vi "process.vi"(8 "error in":errorcluster, 11 "Data.PG":refnum<class "LV-Data.PGSQL.lvclass">) -> ()   [LabVIEW 2019, in "PGC2D.lvlib"]
uses:
  PGC2D.lvlib
  <userlib>/LevyLab/LV-Data/LV-Data.PG/LV-Data.PGSQL.lvclass
  sandbox/Instrument.AML.GetAll--Cluster.ctl
  typedefs/Instrument.AML.PGC2D_Chamber_ID--cluster.ctl
panel:
  in  "Log Fast":bool
  out "Prep Status 2":string caption="Status"
  out "Waveform Chart 2":dbl(graph)
  out "Waveform Chart":dbl(graph)
  out "Prep Current (A)":dbl=4.0 caption="Current (A)"
  out "Analysis Current (A)":dbl=2.0 caption="Current (A)"
  out "Prep Pirani (mbar) 1":dbl=7.0 caption="Pirani 1 (mbar)"
  out "Prep Pirani (mbar) 2":dbl=8.0 caption="Pirani 2 (mbar)"
  out "Analysis Pirani (mbar) 2":dbl=6.0 caption="Pirani 2 (mbar)"
  out "Analysis Pirani (mbar) 1":dbl=5.0 caption="Pirani 1 (mbar)"
  out "Prep Status":string caption="Status"
  out "Analysis Status":string caption="Status"
  out "state":string
  out "logger timer (ms)":u32
  out "Prep Pressure (mbar)":dbl=3.0 caption="IG (mbar)" format="%_2g"
  out "Analysis Pressure (mbar)":dbl=1.0 caption="IG (mbar)" format="%_2g"
  out "Data.PG out":refnum<class "LV-Data.PGSQL.lvclass">
  out "read timer (ms)":u32
  out "error out":errorcluster
  # "Analysis Chamber"
  # "Preparation Chamber"
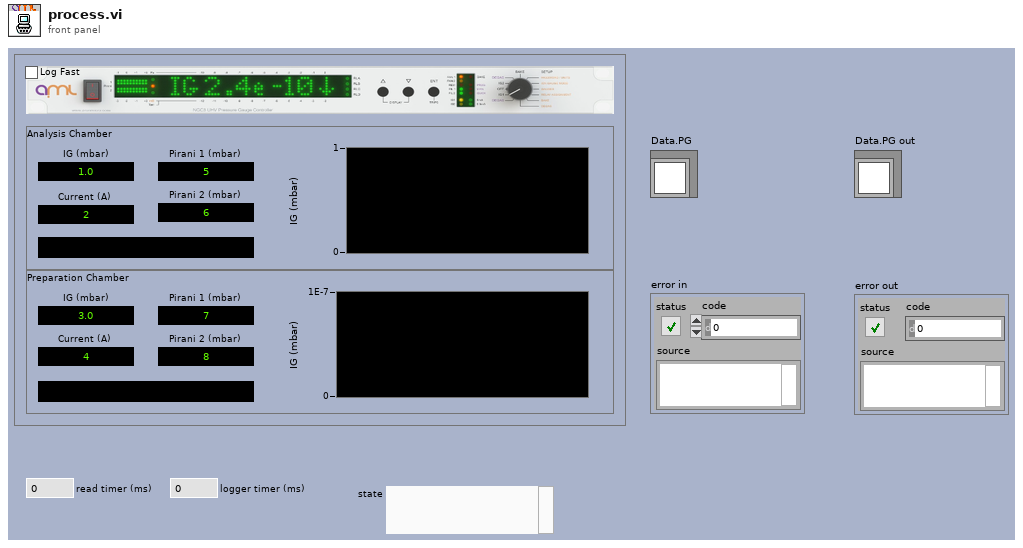
[diagram p1: front panel]
types:
  T1 = enum32{"Invalid", "Standard", "Closed", "Hidden", "Minimized", "Maximized"}
  T2 = enum32{"invalid app kind", "Development System", "Run Time System", "Student Edition", "Embedded LabVIEW", "Evaluation", "Custom"}
  T3 = typedef "PGC2D.lvlib/Instrument.AML.PGC2D_Chamber_ID--cluster.ctl" = cluster{"name":string, "Address":refnum<visa-resource-name>}
  T4 = typedef "Instrument.AML.GetAll--Cluster.ctl" = cluster{"IG Pressure (mbar)":dbl, "Pirani 1 Pressure (mbar)":dbl, "Pirani 2 Pressure (mbar)":dbl, "Emission Current (A)":dbl, "Trip A Pressure (mbar)":dbl, "Trip B Pressure (mbar)":dbl, "Trip C Pressure (mbar)":dbl, "Trip D Pressure (mbar)":dbl, "Instrument Status":string, "Fault":string, "Trip A Association":string, "Trip B Association":string, "Trip C Association":string, "Trip D Association":string, "Relay A":string, "Relay B":string, "Relay C":string, "Relay D":string}
  T5 = cluster{"Core":cluster{"Current VI Reference":refnum<vi>, "Close Panel on Exit?":bool}, "Data.PG":refnum<class "LV-Data.PGSQL.lvclass">, "Chamber ID":T3[], "AML cluster array":T4[]}
  T6 = cluster{"Current VI Reference":refnum<vi>, "Close Panel on Exit?":bool}
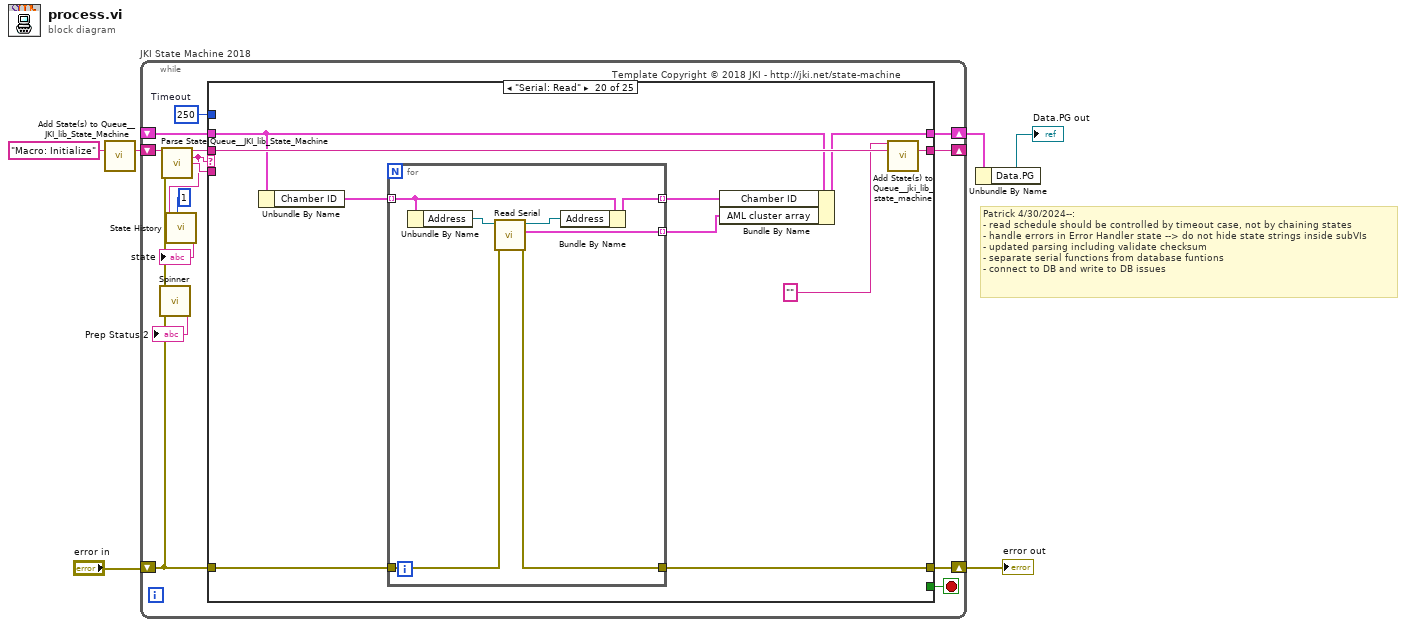
[diagram p0: block diagram]
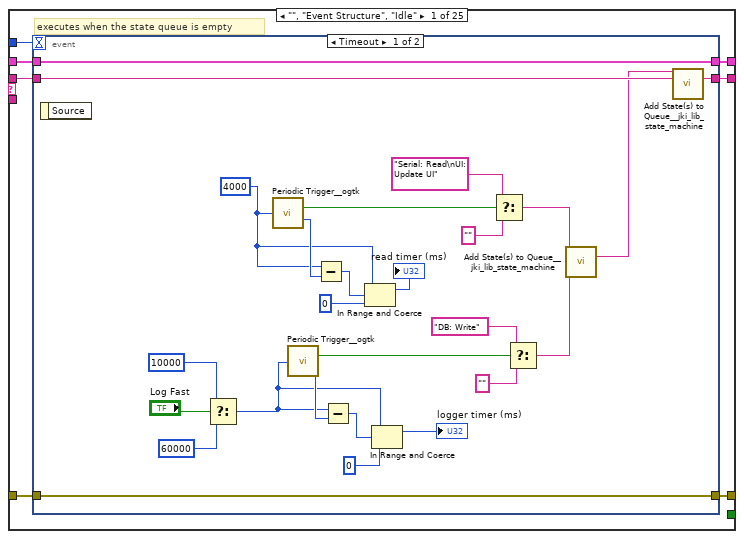
[diagram p2: hidden frame]
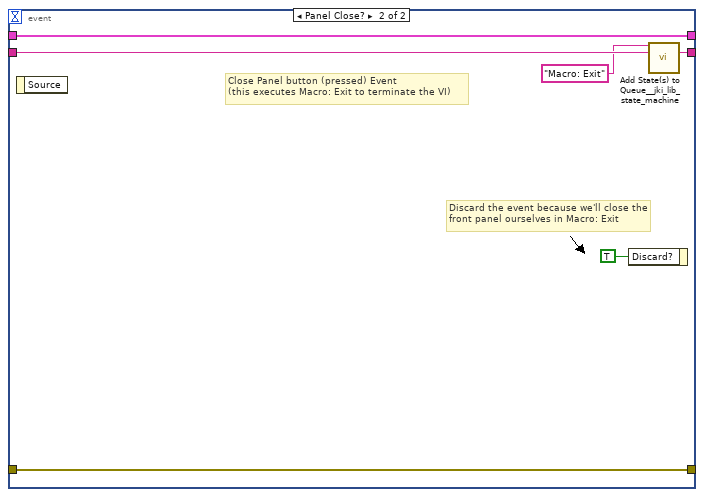
[diagram p3: hidden frame]
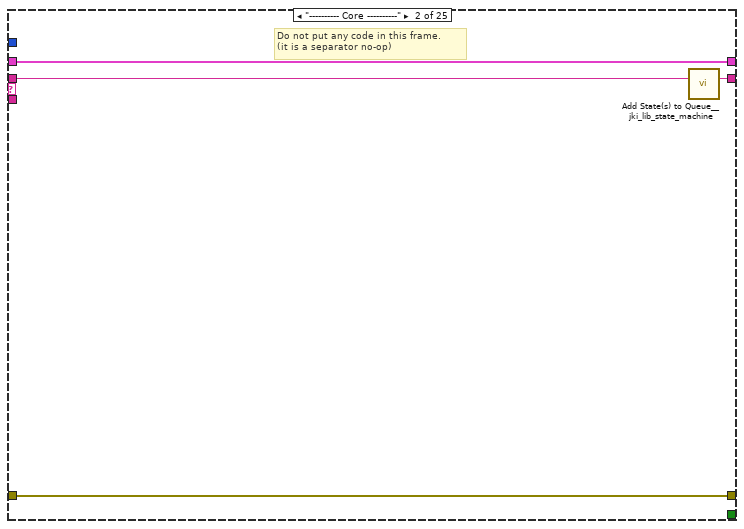
[diagram p4: hidden frame]
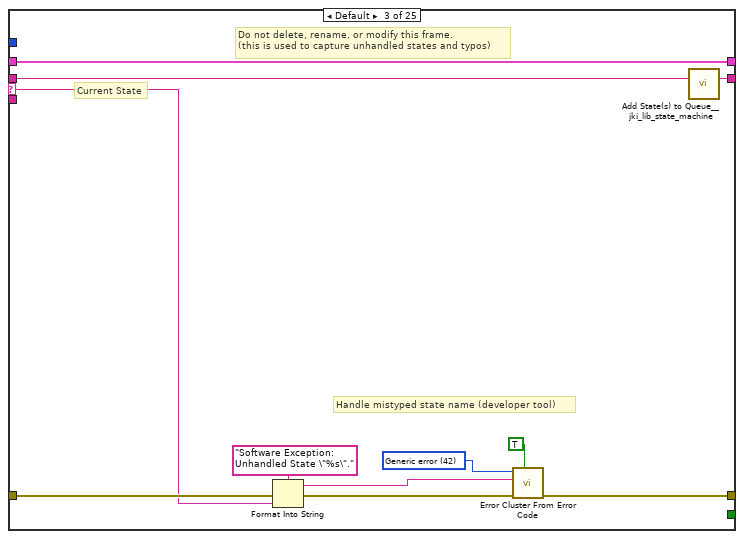
[diagram p5: hidden frame]
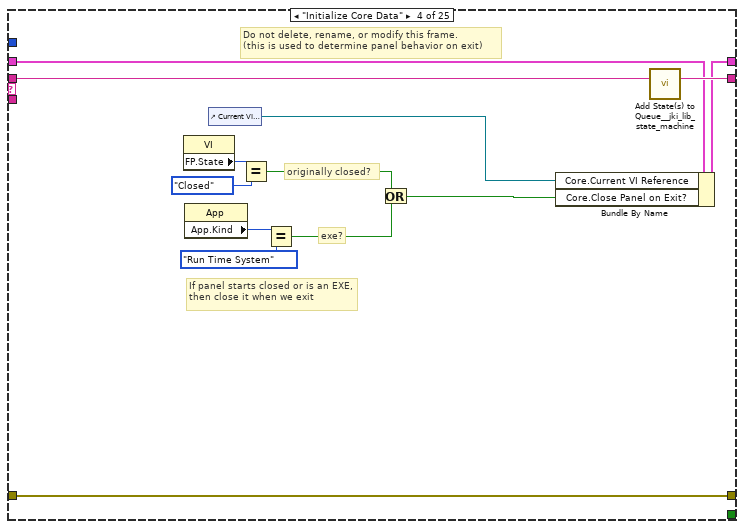
[diagram p6: hidden frame]
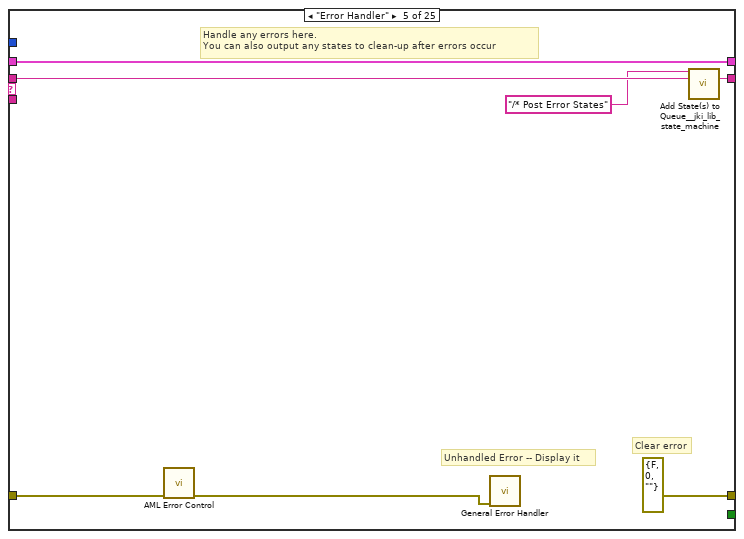
[diagram p7: hidden frame]
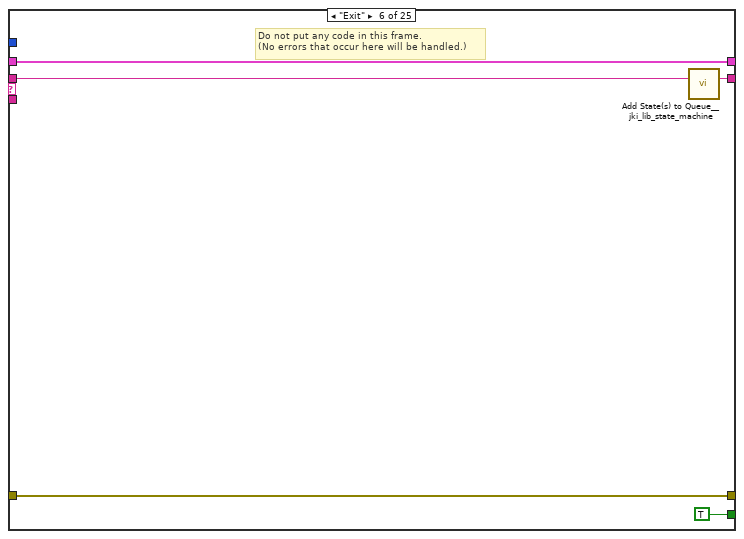
[diagram p8: hidden frame]
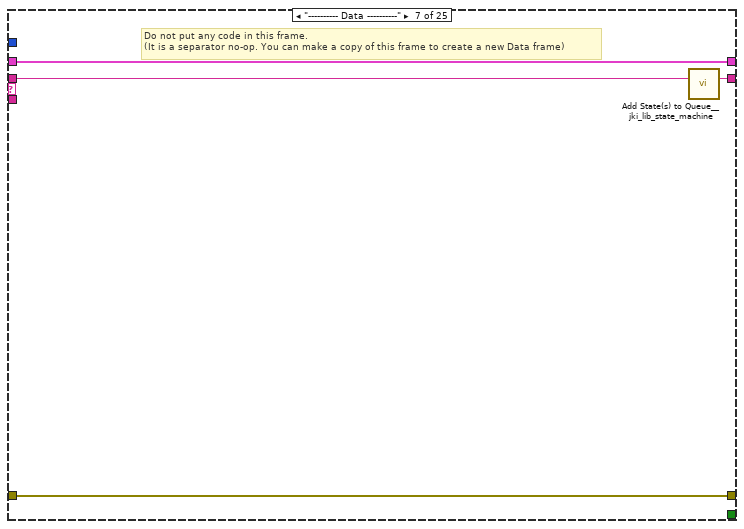
[diagram p9: hidden frame]
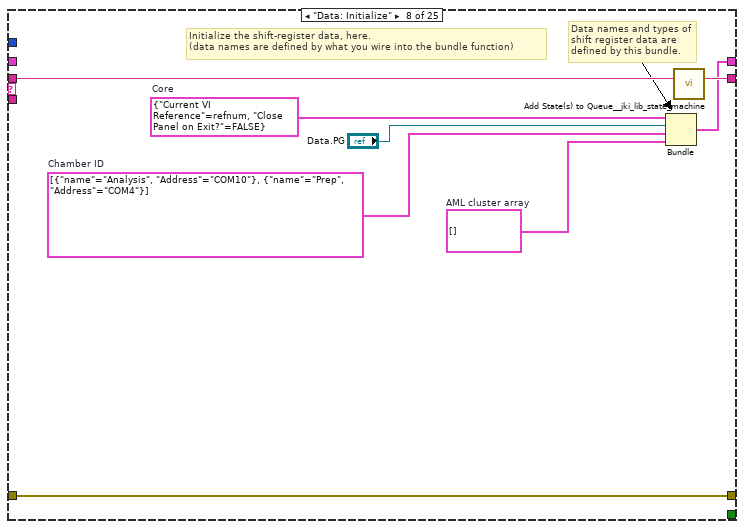
[diagram p10: hidden frame]
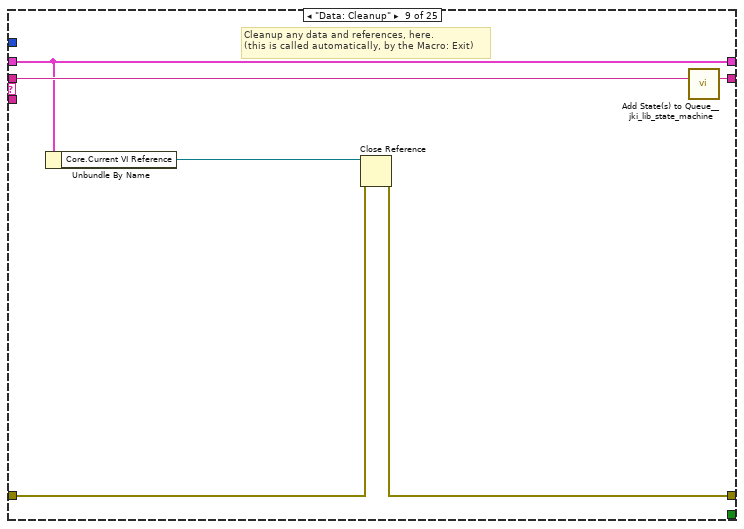
[diagram p11: hidden frame]
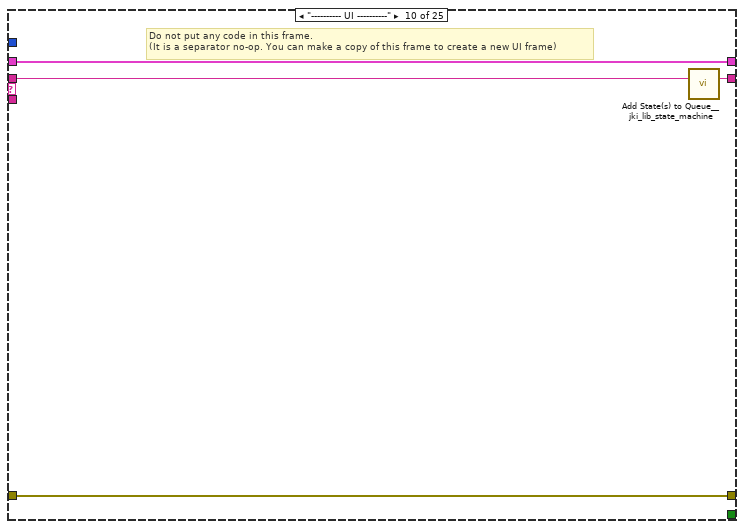
[diagram p12: hidden frame]
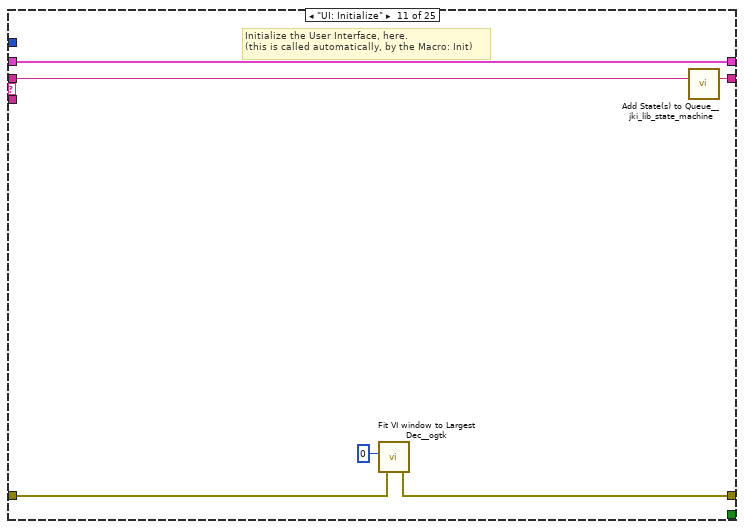
[diagram p13: hidden frame]
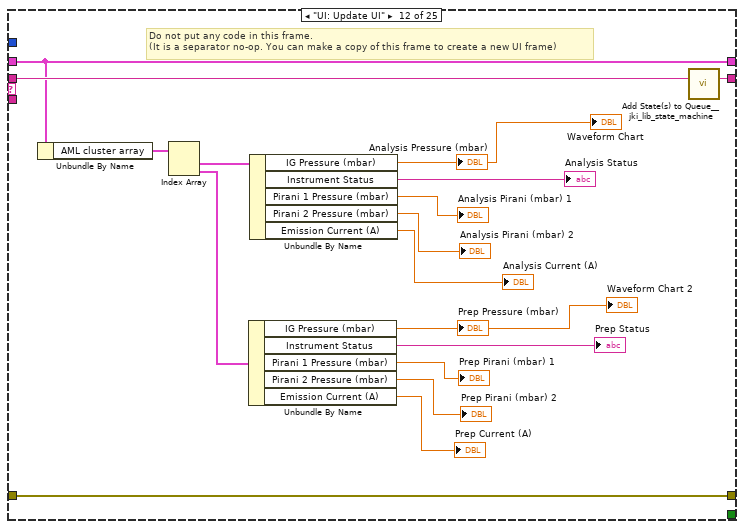
[diagram p14: hidden frame]
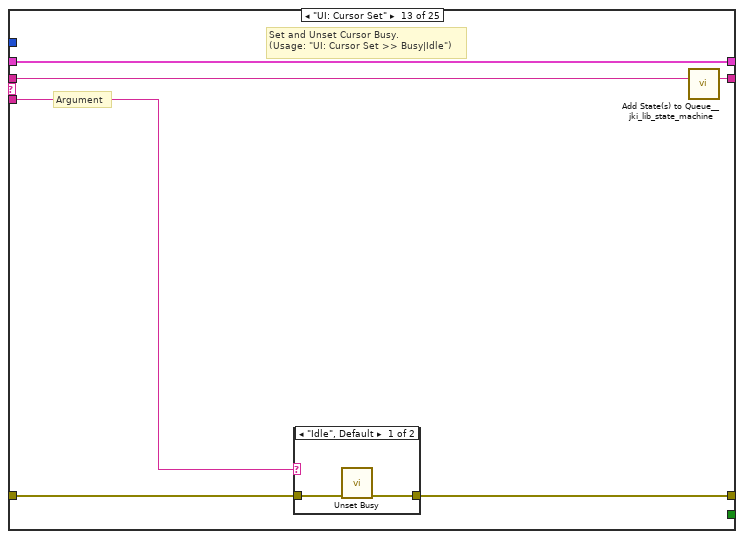
[diagram p15: hidden frame]
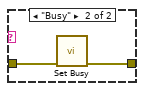
[diagram p16: hidden frame]
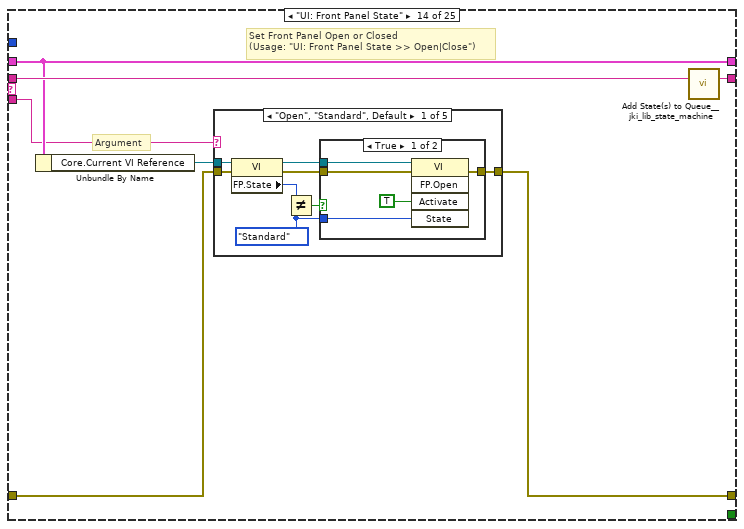
[diagram p17: hidden frame]
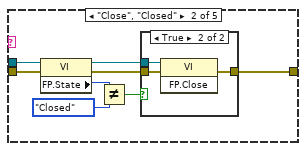
[diagram p19: hidden frame]
diagram:
  # "Patrick 4/30/2024--:\n- read schedule should be controlled by timeout case, not by chaining states\n- handle errors in Error Handler state --> do not hide state strings inside subVIs\n- updated parsing including validate checksum\n- separate serial functions from database funtions\n- connect to DB and write to DB issues"
  n1 = call <vilib>:"Add State(s) to Queue__JKI_lib_State_Machine.vi"("State(s) in (\"\")"="Macro: Initialize") -> ("States Out"=w6:string)  [unwired: 14 in]
  n2 = while "JKI State Machine 2018" {
    shift-right: [w14] -> w2
    shift-left: _ -> [w13]
    shift-right: [w17] -> w4
    shift-left: "error in" -> [w11]
    shift-right: [w16] -> _
    shift-left: w6 -> [w18]
    stop <- w15 stop-if-true
    w12 = 250  # Timeout
    # "Template Copyright © 2018 JKI - http://jki.net/state-machine"
    n3 = call "Spinner.vi"() -> ("element"=→"Prep Status 2":string)  [unwired: 11 in]
    n4 = call <vilib>:"Parse State Queue__JKI_lib_State_Machine.vi"("State Queue"=w18, "Error In (no error)"=w11) -> ("Remaining States"=w20:string, "Current State"=w9:string, "Arguments"=w19:string)  [unwired: 11 in]
    n5 = call "State History.vi"("history length (100)"=1, "Current State"=w9) -> ("History"=→"state":string)  [unwired: 9 in]
    n6 = case shown="\"Serial: Read\"" w9 {
      selector: w9 -> [_ _ w64 _ _ _ _ _ _ _ _ _ _ _ _ _ _ _ _ _ _ _ _ _ _]
      tunnel: w20 -> [w27 w63 w68 w87 w94 w99 w103 w111 w117 w121 w127 w144 w150 w161 w230 w235 w246 w250 w258 w274 w285 w295 w303 w308 w321]
      tunnel: w19 -> [_ _ _ _ _ _ _ _ _ _ _ _ w145 w155 _ _ _ _ _ _ _ _ _ _ _]
      tunnel: w13 -> [w25 w60 w66 w80 w88 w97 w100 _ w112 w118 w125 w141 w148 w157 w227 w232 w243 w247 w256 w267 w282 w292 w298 w305 w317]
      tunnel: [w24 w61 w70 w84 errorcluster {"status"=FALSE, "code"=0, "source"=""} ("error out") w96 w101 w108 w114 w119 w124 w142 w146 w158 w228 w233 w244 w248 w255 w266 w283 w293 w297 w311 w315] -> w17
      tunnel: w11 -> [w23 w61 w69 w84 w90 w96 w101 w108 w113 w119 w123 w142 w147 w159 w228 w233 w244 w248 w253 w270 w284 w293 w296 w312 w314]
      tunnel: [w26 w62 w67 w86 w93 w98 w102 w110 w116 w120 w126 w143 w149 w160 w229 w234 w245 w249 w257 w273 w286 w294 w302 w309 w320] -> w16
      tunnel: [_ _ _ _ _ TRUE _ _ _ _ _ _ _ _ _ _ _ _ _ _ _ _ _ _ _] -> w15
      tunnel: [w22 w60 w66 w85 w88 w97 w100 w109 w112 w118 w125 w141 w148 w157 w227 w232 w243 w247 w252 w268 w282 w292 w299 w307 w318] -> w14
      tunnel: w12 -> [w21 _ _ _ _ _ _ _ _ _ _ _ _ _ _ _ _ _ _ _ _ _ _ _ _]
      frame "", "Event Structure", "Idle" {
        # "executes when the state queue is empty"
        n7 = event shown="[0] Timeout" {
          selector: _ -> [_ _]
          dyn-events: _ -> [_ _]
          timeout: w21 -> [_ _]
          tunnel: w27 -> [w53 w59]
          tunnel: [w52 w58] -> w26
          tunnel: w25 -> [w50 w56]
          tunnel: [w51 w57] -> w24
          tunnel: w23 -> [w51 w57]
          tunnel: [w50 w56] -> w22
          event Timeout {
            w36 = u32 4000 ("wait (ms)")
            n8 = event-data() -> ()  [unwired: 1 in, 1 out]
            n9 = Select(t=u32 10000, s="Log Fast", f=u32 60000 ("time (ms)")) -> (s? t:f=w30:u32)
            n10 = call <userlib>:"Periodic Trigger__ogtk.vi"("time (ms)"=w36) -> ("Triggered"=w48:bool, "timer value"=w49:u32)  [unwired: 12 in, 1 out]
            n11 = call <userlib>:"Periodic Trigger__ogtk.vi"("time (ms)"=w30) -> ("Triggered"=w42:bool, "timer value"=w34:u32)  [unwired: 12 in, 1 out]
            n12 = Subtract(x=w36, y=w49) -> (x-y=w38:u32)
            n13 = Subtract(x=w30, y=w34) -> (x-y=w35:u32)
            n14 = In Range and Coerce(upper limit=w36, x=w38, lower limit=u32 0) -> (coerced(x)=→"read timer (ms)":u32)  [unwired: 1 out]
            n15 = In Range and Coerce(upper limit=w30, x=w35, lower limit=u32 0) -> (coerced(x)=→"logger timer (ms)":u32)  [unwired: 1 out]
            n16 = Select(t="Serial: Read\nUI: Update UI" ("State(s) in Front (\"\")"), s=w48, f="" ("State(s) in Front (\"\")")) -> (s? t:f=w45:string)
            n17 = Select(t="DB: Write" ("State(s) in Front (\"\")"), s=w42, f="" ("State(s) in Front (\"\")")) -> (s? t:f=w41:string)
            n18 = call <vilib>:"Add State(s) to Queue__jki_lib_state_machine.vi"("State(s) in Front (\"\")"=w45, "State(s) at Back (\"\")"=w41) -> ("States Out"=w40:string)  [unwired: 13 in]
            n19 = call <vilib>:"Add State(s) to Queue__jki_lib_state_machine.vi"("State(s) in Front (\"\")"=w40, "State(s) in (\"\")"=w53) -> ("States Out"=w52:string)  [unwired: 13 in]
          }
          event Panel Close? {
            # "Discard the event because we'll close the front panel ourselves in Macro: Exit"
            # "Close Panel button (pressed) Event\n(this executes Macro: Exit to terminate the VI)"
            n20 = event-data() -> ()  [unwired: 1 in, 1 out]
            n21 = event-data("Discard?"=TRUE) -> ()  [unwired: 1 in, 1 out]
            n22 = call <vilib>:"Add State(s) to Queue__jki_lib_state_machine.vi"("State(s) in Front (\"\")"="Macro: Exit", "State(s) in (\"\")"=w59) -> ("States Out"=w58:string)  [unwired: 13 in]
          }
        }
      }
      frame "---------- Core ----------" {
        # "Do not put any code in this frame.\n(it is a separator no-op)"
        n23 = call <vilib>:"Add State(s) to Queue__jki_lib_state_machine.vi"("State(s) in (\"\")"=w63) -> ("States Out"=w62:string)  [unwired: 14 in]
      }
      frame Default {
        w73 = 42 items=["No error", "Argument error", "Memory is full", "Out of zone", "End of file", "File already open", "Generic file I/O error", "File not found", "File permission error", "Disk is full", "Duplicate path", "Too many files open", "System feature not enabled", "Resource file not found", "Cannot add resource", "Resource not found", "Image not found", "Image memory error", "Pen does not exist", "Config type invalid", "Config token not found", "Config parse error", "Config memory error", "Bad external code format", "Bad external code offset", "External code not present", "Null window", "Destroy window error", "Null menu", "Print aborted", "Bad print record", "Print driver error", "Windows error during printing", "Memory error during printing", "Print dialog error", "Generic print error", "Invalid device refnum", "Device not found", "Device parameter error", "Device unit error", "Cannot open device", "Device call aborted", "Generic error", "Cancelled by user", "Object ID too low", "Object ID too high", "Object not in heap", "Unknown heap", "Unknown object (invalid DefProc)", "Unknown object (DefProc not in table)", "Message out of range", "Invalid (null) method", "Unknown message", "Manager call not supported", "Bad address", "Network operation in progress", "Network operation timed out", "Connection is busy", "Network attribute not supported", "Network error", "Address in use", "System out of memory", "Connection aborted", "Connection refused", "Not connected", "Already connected", "Connection closed", "Initialization error (interapplication manager)", "Bad occurrence", "Wait on unbound occurrence handler", "Occurrence queue overflow", "Datalog type conflict", "Unused", "Unrecognized type (interapplication manager)", "Memory corrupt", "Failed to make temporary DLL", "Old CIN version", "Drag socket not found", "Failed to load drop-object", "Failed to register OLE object", "Failed to release OLE object", "Format specifier type mismatch", "Unknown format specifier", "Too few format specifiers", "Too many format specifiers", "Scan failed", "Newer CIN version", "Error converting to variant", "Runtime menu error", "Password tampered", "Variant attribute not found", "Incompatible variant data type", "Event data is not available", "Event Store is not present", "Occurrence is not found", "Event Queue is not created", "Event info is not available", "Refnum passed is NULL", "Error retrieving Class GUID", "Error retrieving CoClass GUID", "Error retrieving TypeLib GUID.", "Bad built application magic bytes.", "Specific driver is different from the specific driver associated with the Logical Name.", "There is no session opened to the class driver.", "Max Error", "MAX - Error with config objects", "MAX - Error loading configuration", "MAX - Group not supported"]
        # "Current State"
        # "Do not delete, rename, or modify this frame.\n(this is used to capture unhandled states and typos)"
        # "Handle mistyped state name (developer tool)"
        n24 = Format Into String(format string="Software Exception: Unhandled State \"%s\"." ("message"), error in=w69, w64) -> (resulting string=w72:string, error out=w71:errorcluster)  [unwired: 1 in]
        n25 = call <vilib>:"Error Cluster From Error Code.vi"("show call chain? (False)"=TRUE, "error in (no error)"=w71, "error message (\"\")"=w72, "error code (0)"=w73) -> ("error out"=w70:errorcluster)  [unwired: 5 in]
        n26 = call <vilib>:"Add State(s) to Queue__jki_lib_state_machine.vi"("State(s) in (\"\")"=w68) -> ("States Out"=w67:string)  [unwired: 14 in]
      }
      frame "Initialize Core Data" {
        # "Do not delete, rename, or modify this frame.\n(this is used to determine panel behavior on exit)"
        # "originally closed?"
        # "exe?"
        # "If panel starts closed or is an EXE, then close it when we exit"
        n27 = property class="VI"() -> ("FP.State"=w77:T1)  [unwired: 2 in, 2 out]
        n28 = property class="App"() -> ("App.Kind"=w83:T2)  [unwired: 2 in, 2 out]
        n29 = control-ref of="Current VI Reference"() -> (w78:refnum<vi>)
        n30 = Equal?(x=w77, y=T1."Closed" ("Front Panel Window:State")) -> (x = y?=w75:bool)
        n31 = Equal?(x=w83, y=T2."Run Time System" ("Application:Kind")) -> (x = y?=w81:bool)
        n32 = Or(x=w75, y=w81) -> (x .or. y?=w79:bool)
        n33 = Bundle By Name(cluster=w80, "Core.Current VI Reference"=w78, "Core.Close Panel on Exit?"=w79) -> (w85:T5)
        n34 = call <vilib>:"Add State(s) to Queue__jki_lib_state_machine.vi"("State(s) in (\"\")"=w87) -> ("States Out"=w86:string)  [unwired: 14 in]
      }
      frame "Error Handler" {
        # "Unhandled Error -- Display it"
        # "Handle any errors here.\nYou can also output any states to clean-up after errors occur"
        # "Clear error"
        n35 = call "AML Error Control.vi"("input cluster"=w90) -> ("error out"=w89:errorcluster)  [unwired: 8 in, 2 out]
        n36 = call <vilib>:"General Error Handler.vi"("error in (no error)"=w89) -> ()  [unwired: 10 in, 5 out]
        n37 = call <vilib>:"Add State(s) to Queue__jki_lib_state_machine.vi"("State(s) in Front (\"\")"="/* Post Error States", "State(s) in (\"\")"=w94) -> ("States Out"=w93:string)  [unwired: 13 in]
      }
      frame "Exit" {
        # "Do not put any code in this frame.\n(No errors that occur here will be handled.)"
        n38 = call <vilib>:"Add State(s) to Queue__jki_lib_state_machine.vi"("State(s) in (\"\")"=w99) -> ("States Out"=w98:string)  [unwired: 14 in]
      }
      frame "---------- Data ----------" {
        # "Do not put any code in this frame.\n(It is a separator no-op. You can make a copy of this frame to create a new Data frame)"
        n39 = call <vilib>:"Add State(s) to Queue__jki_lib_state_machine.vi"("State(s) in (\"\")"=w103) -> ("States Out"=w102:string)  [unwired: 14 in]
      }
      frame "Data: Initialize" {
        w105 = T3[] [{"name"="Analysis", "Address"="COM10"}, {"name"="Prep", "Address"="COM4"}]  # Chamber ID
        w106 = T4[] []  # AML cluster array
        w107 = T6 {"Current VI Reference"=refnum, "Close Panel on Exit?"=FALSE}  # Core
        # "Data names and types of shift register data are defined by this bundle."
        # "Initialize the shift-register data, here.\n(data names are defined by what you wire into the bundle function)"
        n40 = Bundle("Core"=w107, "Data.PG"="Data.PG", "Chamber ID"=w105, "AML cluster array"=w106) -> (w109:T5)  [unwired: 1 in]
        n41 = call <vilib>:"Add State(s) to Queue__jki_lib_state_machine.vi"("State(s) in (\"\")"=w111) -> ("States Out"=w110:string)  [unwired: 14 in]
      }
      frame "Data: Cleanup" {
        # "Cleanup any data and references, here.\n(this is called automatically, by the Macro: Exit)"
        n42 = Unbundle By Name(w112) -> ("Core.Current VI Reference"=w115:refnum<vi>)
        n43 = Close Reference(reference=w115, error in (no error)=w113) -> (error out=w114:errorcluster)
        n44 = call <vilib>:"Add State(s) to Queue__jki_lib_state_machine.vi"("State(s) in (\"\")"=w117) -> ("States Out"=w116:string)  [unwired: 14 in]
      }
      frame "---------- UI ----------" {
        # "Do not put any code in this frame.\n(It is a separator no-op. You can make a copy of this frame to create a new UI frame)"
        n45 = call <vilib>:"Add State(s) to Queue__jki_lib_state_machine.vi"("State(s) in (\"\")"=w121) -> ("States Out"=w120:string)  [unwired: 14 in]
      }
      frame "UI: Initialize" {
        # "Initialize the User Interface, here.\n(this is called automatically, by the Macro: Init)"
        n46 = call <userlib>:"Fit VI window to Largest Dec__ogtk.vi"("error in (no error)"=w123, "border spacing (2 px)"=0) -> ("error out"=w124:errorcluster)  [unwired: 4 in, 1 out]
        n47 = call <vilib>:"Add State(s) to Queue__jki_lib_state_machine.vi"("State(s) in (\"\")"=w127) -> ("States Out"=w126:string)  [unwired: 14 in]
      }
      frame "UI: Update UI" {
        # "Do not put any code in this frame.\n(It is a separator no-op. You can make a copy of this frame to create a new UI frame)"
        n48 = Unbundle By Name(w141) -> ("AML cluster array"=w140:T4[])
        n49 = Index Array(array=w140) -> (element #1=w139:T4, element #2=w136:T4)  [unwired: 2 in]
        n50 = Unbundle By Name(w136) -> ("IG Pressure (mbar)"=→"Prep Pressure (mbar)" →"Waveform Chart 2":dbl, "Instrument Status"=→"Prep Status":string, "Pirani 1 Pressure (mbar)"=→"Prep Pirani (mbar) 1":dbl, "Pirani 2 Pressure (mbar)"=→"Prep Pirani (mbar) 2":dbl, "Emission Current (A)"=→"Prep Current (A)":dbl)
        n51 = Unbundle By Name(w139) -> ("IG Pressure (mbar)"=→"Analysis Pressure (mbar)" →"Waveform Chart":dbl, "Instrument Status"=→"Analysis Status":string, "Pirani 1 Pressure (mbar)"=→"Analysis Pirani (mbar) 1":dbl, "Pirani 2 Pressure (mbar)"=→"Analysis Pirani (mbar) 2":dbl, "Emission Current (A)"=→"Analysis Current (A)":dbl)
        n52 = call <vilib>:"Add State(s) to Queue__jki_lib_state_machine.vi"("State(s) in (\"\")"=w144) -> ("States Out"=w143:string)  [unwired: 14 in]
      }
      frame "UI: Cursor Set" {
        # "Argument"
        # "Set and Unset Cursor Busy.\n(Usage: \"UI: Cursor Set >> Busy|Idle\")"
        n53 = case shown="\"Idle\", Default" w145 {
          tunnel: w147 -> [w152 w154]
          tunnel: [w151 w153] -> w146
          frame "Idle", Default {
            n54 = call <vilib>:"Unset Busy.vi"("error in (no error)"=w152) -> ("error out"=w151:errorcluster)  [unwired: 10 in]
          }
          frame "Busy" {
            n55 = call <vilib>:"Set Busy.vi"("error in (no error)"=w154) -> ("error out"=w153:errorcluster)  [unwired: 9 in, 1 out]
          }
        }
        n56 = call <vilib>:"Add State(s) to Queue__jki_lib_state_machine.vi"("State(s) in (\"\")"=w150) -> ("States Out"=w149:string)  [unwired: 14 in]
      }
      frame "UI: Front Panel State" {
        # "Argument"
        # "Set Front Panel Open or Closed\n(Usage: \"UI: Front Panel State >> Open|Close\")"
        n57 = Unbundle By Name(w157) -> ("Core.Current VI Reference"=w156:refnum<vi>)
        n58 = case shown="\"Open\", \"Standard\", Default" w155 {
          tunnel: w159 -> [w167 w182 w193 w206 w219]
          tunnel: [w169 w183 w195 w208 w221] -> w158
          tunnel: w156 -> [w168 w180 w194 w207 w220]
          frame "Open", "Standard", Default {
            w162 = T1."Standard" ("State")
            n59 = property class="VI"(reference=w168, error in=w167) -> (reference out=w165:refnum<vi>, error out=w166:errorcluster, "FP.State"=w164:T1)
            n60 = Not Equal?(x=w164, y=w162) -> (x != y?=w163:bool)
            n61 = case shown="True" w163 {
              tunnel: [w173 w175] -> w169
              tunnel: w166 -> [w172 w175]
              tunnel: w165 -> [w171 _]
              tunnel: w162 -> [w170 _]
              frame True {
                n62 = invoke class="VI" method="FP.Open"(reference=w171, error in=w172, "Activate"=TRUE, "State"=w170) -> (error out=w173:errorcluster)  [unwired: 1 in, 4 out]
              }
              frame False {
              }
            }
          }
          frame "Close", "Closed" {
            n63 = property class="VI"(reference=w180, error in=w182) -> (reference out=w179:refnum<vi>, error out=w181:errorcluster, "FP.State"=w177:T1)
            n64 = Not Equal?(x=w177, y=T1."Closed" ("Front Panel Window:State")) -> (x != y?=w176:bool)
            n65 = case shown="True" w176 {
              tunnel: [w184 w187] -> w183
              tunnel: w181 -> [w184 w186]
              tunnel: w179 -> [_ w185]
              frame False {
              }
              frame True {
                n66 = invoke class="VI" method="FP.Close"(reference=w185, error in=w186) -> (error out=w187:errorcluster)  [unwired: 1 in, 2 out]
              }
            }
          }
          frame "Hidden", "Hide" {
            w188 = T1."Hidden" ("State")
            n67 = property class="VI"(reference=w194, error in=w193) -> (reference out=w191:refnum<vi>, error out=w192:errorcluster, "FP.State"=w190:T1)
            n68 = Not Equal?(x=w190, y=w188) -> (x != y?=w189:bool)
            n69 = case shown="True" w189 {
              tunnel: [w199 w200] -> w195
              tunnel: w192 -> [w198 w200]
              tunnel: w191 -> [w197 _]
              tunnel: w188 -> [w196 _]
              frame True {
                n70 = invoke class="VI" method="FP.Open"(reference=w197, error in=w198, "State"=w196) -> (error out=w199:errorcluster)  [unwired: 2 in, 4 out]
              }
              frame False {
              }
            }
          }
          frame "Minimize", "Minimized" {
            w201 = T1."Minimized" ("State")
            n71 = property class="VI"(reference=w207, error in=w206) -> (reference out=w204:refnum<vi>, error out=w205:errorcluster, "FP.State"=w203:T1)
            n72 = Not Equal?(x=w203, y=w201) -> (x != y?=w202:bool)
            n73 = case shown="True" w202 {
              tunnel: [w212 w213] -> w208
              tunnel: w205 -> [w211 w213]
              tunnel: w204 -> [w210 _]
              tunnel: w201 -> [w209 _]
              frame True {
                n74 = invoke class="VI" method="FP.Open"(reference=w210, error in=w211, "State"=w209) -> (error out=w212:errorcluster)  [unwired: 2 in, 4 out]
              }
              frame False {
              }
            }
          }
          frame "Maximize", "Maximized" {
            w214 = T1."Maximized" ("State")
            n75 = property class="VI"(reference=w220, error in=w219) -> (reference out=w217:refnum<vi>, error out=w218:errorcluster, "FP.State"=w216:T1)
            n76 = Not Equal?(x=w216, y=w214) -> (x != y?=w215:bool)
            n77 = case shown="True" w215 {
              tunnel: [w225 w226] -> w221
              tunnel: w218 -> [w224 w226]
              tunnel: w217 -> [w223 _]
              tunnel: w214 -> [w222 _]
              frame True {
                n78 = invoke class="VI" method="FP.Open"(reference=w223, error in=w224, "State"=w222) -> (error out=w225:errorcluster)  [unwired: 2 in, 4 out]
              }
              frame False {
              }
            }
          }
        }
        n79 = call <vilib>:"Add State(s) to Queue__jki_lib_state_machine.vi"("State(s) in (\"\")"=w161) -> ("States Out"=w160:string)  [unwired: 14 in]
      }
      frame "---------- Macro ----------" {
        # "Do not put any code in this frame.\n(It is a separator no-op. You can make a copy of this frame to create a new Macro frame)"
        n80 = call <vilib>:"Add State(s) to Queue__jki_lib_state_machine.vi"("State(s) in (\"\")"=w230) -> ("States Out"=w229:string)  [unwired: 14 in]
      }
      frame "Macro: Initialize" {
        w231 = "Data: Initialize\nInitialize Core Data\nUI: Initialize\nUI: Front Panel State >> Open\n\nDB: Connect\nSerial: Initialize\nSerial: Read\nUI: Update UI"  # Data: Initialize Initialize Core Data UI: Initialize UI: Front Panel State >> Open  DB: Connect Serial: Initialize Serial: Read UI: Update UI
        # "Initialization Macro\n(This is called once, when the VI starts)"
        n81 = call <vilib>:"Add State(s) to Queue__jki_lib_state_machine.vi"("State(s) in Front (\"\")"=w231, "State(s) in (\"\")"=w235) -> ("States Out"=w234:string)  [unwired: 13 in]
      }
      frame "Macro: Exit" {
        # "Exit Macro\n(This is called once, when the VI exits)"
        n82 = Unbundle By Name(w243) -> ("Core.Close Panel on Exit?"=w242:bool)
        n83 = Select(t="UI: Front Panel State >> Close", s=w242, f="") -> (s? t:f=w239:string)
        n84 = call <vilib>:"Add State(s) to Queue__jki_lib_state_machine.vi"("State(s) in Front (\"\")"="Serial: Close\nDB: Disconnect", "State(s) in (\"\")"=w239, "State(s) at Back (\"\")"="Data: Cleanup\nExit") -> ("States Out"=w237:string)  [unwired: 12 in]
        n85 = call <vilib>:"Add State(s) to Queue__jki_lib_state_machine.vi"("State(s) in Front (\"\")"=w237, "State(s) in (\"\")"=w246) -> ("States Out"=w245:string)  [unwired: 13 in]
      }
      frame "---------- Serial ----------" {
        # "Template Separator\n(You can make a copy of, or modify, this frame)"
        n86 = call <vilib>:"Add State(s) to Queue__jki_lib_state_machine.vi"("State(s) in (\"\")"=w250) -> ("States Out"=w249:string)  [unwired: 14 in]
      }
      frame "Serial: Initialize" {
        n87 = Unbundle By Name(w256) -> ("Chamber ID"=w254:T3[])
        n88 = for {
          tunnel: w254 -> [w259] mode=indexing
          tunnel: w253 -> [w264]
          tunnel: [w263] -> w255
          tunnel: [w260] -> w251 mode=indexing
          n89 = Unbundle By Name(w259) -> ("Address"=w262:refnum<visa-resource-name>)
          n90 = call "Initialize Serial.vi"("error in (no error)"=w264, "VISA resource name"=w262) -> ("error out"=w263:errorcluster, "VISA resource name out"=w261:refnum<visa-resource-name>)  [unwired: 8 in]
          n91 = Bundle By Name(cluster=w259, "Address"=w261) -> (w260:T3)
        }
        n92 = Bundle By Name(cluster=w256, "Chamber ID"=w251) -> (w252:T5)
        n93 = call <vilib>:"Add State(s) to Queue__jki_lib_state_machine.vi"("State(s) in (\"\")"=w258) -> ("States Out"=w257:string)  [unwired: 14 in]
      }
      frame "Serial: Read" {
        n94 = Unbundle By Name(w267) -> ("Chamber ID"=w271:T3[])
        n95 = for {
          tunnel: [w275] -> w272 mode=indexing
          tunnel: w271 -> [w276] mode=indexing
          tunnel: [w281] -> w265 mode=indexing
          tunnel: w270 -> [w279]
          tunnel: [w280] -> w266
          n96 = Unbundle By Name(w276) -> ("Address"=w278:refnum<visa-resource-name>)
          n97 = call "Read Serial.vi"("error in (no error)"=w279, "VISA Reference"=w278) -> ("error out"=w280:errorcluster, "GetAll"=w281:T4, "VISA Reference out"=w277:refnum<visa-resource-name>)  [unwired: 7 in]
          n98 = Bundle By Name(cluster=w276, "Address"=w277) -> (w275:T3)
        }
        n99 = Bundle By Name(cluster=w267, "Chamber ID"=w272, "AML cluster array"=w265) -> (w268:T5)
        n100 = call <vilib>:"Add State(s) to Queue__jki_lib_state_machine.vi"("State(s) in Front (\"\")"="", "State(s) in (\"\")"=w274) -> ("States Out"=w273:string)  [unwired: 13 in]
      }
      frame "Serial: Close" {
        n101 = Unbundle By Name(w282) -> ("Chamber ID"=w287:T3[])
        n102 = for {
          tunnel: w287 -> [w288] mode=indexing
          tunnel: w284 -> [w291]
          tunnel: [w290] -> w283
          n103 = Unbundle By Name(w288) -> ("Address"=w289:refnum<visa-resource-name>)
          n104 = call "Close Serial.vi"("error in (no error)"=w291, "VISA Reference"=w289) -> ("error out"=w290:errorcluster)  [unwired: 9 in]
        }
        n105 = call <vilib>:"Add State(s) to Queue__jki_lib_state_machine.vi"("State(s) in (\"\")"=w285) -> ("States Out"=w286:string)  [unwired: 14 in]
      }
      frame "---------- DB ----------" {
        # "Template Separator\n(You can make a copy of, or modify, this frame)"
        n106 = call <vilib>:"Add State(s) to Queue__jki_lib_state_machine.vi"("State(s) in (\"\")"=w295) -> ("States Out"=w294:string)  [unwired: 14 in]
      }
      frame "DB: Connect" {
        # "Template Separator\n(You can make a copy of, or modify, this frame)"
        n107 = Unbundle By Name(w298) -> ("Data.PG"=w301:refnum<class "LV-Data.PGSQL.lvclass">)
        n108 = call <userlib>:"PGSQL.Open.vi"("error in (no error)"=w296, "Data.PG in"=w301) -> ("error out"=w297:errorcluster, "Data.PG out"=w300:refnum<class "LV-Data.PGSQL.lvclass">)  [unwired: 8 in]
        n109 = Bundle By Name(cluster=w298, "Data.PG"=w300) -> (w299:T5)
        n110 = call <vilib>:"Add State(s) to Queue__jki_lib_state_machine.vi"("State(s) in (\"\")"=w303) -> ("States Out"=w302:string)  [unwired: 14 in]
      }
      frame "DB: Write" {
        n111 = Unbundle By Name(w305) -> ("Data.PG"=w313:refnum<class "LV-Data.PGSQL.lvclass">, "AML cluster array"=w306:T4[], "Chamber ID"=w304:T3[])
        n112 = call "Write to DB.vi"("error in"=w312, "Chamber ID"=w304, "AML Cluster const"=w306, "Data.PG in"=w313) -> ("error out"=w311:errorcluster, "Data.PG out"=w310:refnum<class "LV-Data.PGSQL.lvclass">)  [unwired: 5 in, 1 out]
        n113 = Bundle By Name(cluster=w305, "Data.PG"=w310) -> (w307:T5)
        n114 = call <vilib>:"Add State(s) to Queue__jki_lib_state_machine.vi"("State(s) in (\"\")"=w308) -> ("States Out"=w309:string)  [unwired: 14 in]
      }
      frame "DB: Disconnect" {
        # "Template Separator\n(You can make a copy of, or modify, this frame)"
        n115 = Unbundle By Name(w317) -> ("Data.PG"=w316:refnum<class "LV-Data.PGSQL.lvclass">)
        n116 = call-dynamic "Close.vi"("error in (no error)"=w314, "Data.PG in"=w316) -> ("error out"=w315:errorcluster, "Data.PG out"=w319:refnum<class "LV-Data.PGSQL.lvclass">)  [unwired: 8 in]
        n117 = Bundle By Name(cluster=w317, "Data.PG"=w319) -> (w318:T5)
        n118 = call <vilib>:"Add State(s) to Queue__jki_lib_state_machine.vi"("State(s) in (\"\")"=w321) -> ("States Out"=w320:string)  [unwired: 14 in]
      }
    }
  }
  "error out" <- w4
  n119 = Unbundle By Name(w2) -> ("Data.PG"=→"Data.PG out":refnum<class "LV-Data.PGSQL.lvclass">)
